vi "Get Oneof Fields.vi"(8 "error in (no error)":errorcluster, 11 "Message ref in":u64) -> (0 "error out":errorcluster, 2 "Field refs":u64[](array[numeric]), 3 "Message ref out":u64)   [LabVIEW 2019, in "gRPC Template Creation Utility.lvlib"]
uses:
  gRPC Template Creation Utility.lvlib
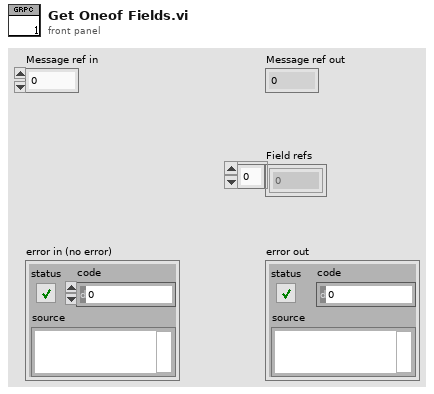
[diagram p1: front panel]
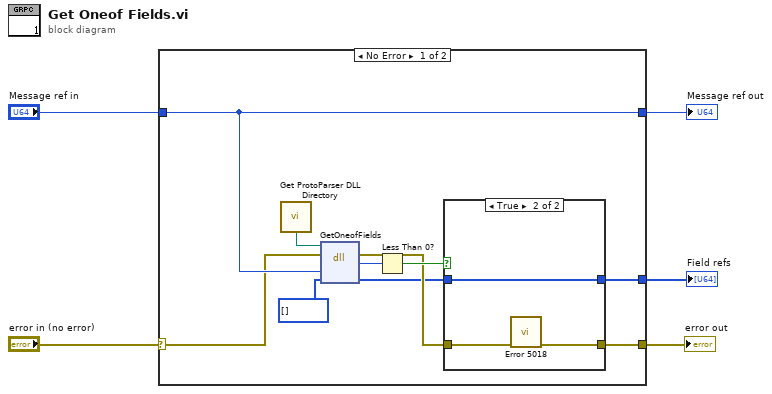
[diagram p0: block diagram]
diagram:
  n1 = case shown="No Error" "error in (no error)" {
    selector: "error in (no error)" -> [w12 w21]
    tunnel: "Message ref in" -> [w13 w22]
    tunnel: [w7 _] -> w4
    tunnel: [w13 w22] -> w3
    tunnel: [w6 w21] -> w1
    frame No Error {
      n2 = call "Get ProtoParser DLL Directory.vi"() -> ("Proto Parser Directory"=w14:path)
      n3 = dll-call lib="C:/Source/grpc-labview/build/Debug/labview_grpc_generator.dll" fn="GetOneofFields"(path in=w14, error in=w12, "message"=w13, "fieldInfo"=u64[] []) -> (error out=w9:errorcluster, "return type"=w11:i32, "fieldInfo"=w8:u64[])  [unwired: 2 in, 1 out]
      n4 = Less Than 0?(x=w11) -> (x < 0?=w10:bool)
      n5 = case shown="True" w10 {
        tunnel: w9 -> [w16 w20]
        tunnel: w8 -> [w17 w19]
        tunnel: [w17 w19] -> w7
        tunnel: [w16 w18] -> w6
        frame False {
        }
        frame True {
          n6 = call "Error 5018.vi"("error in (no error)"=w20) -> ("error out"=w18:errorcluster)  [unwired: 10 in]
        }
      }
    }
    frame Error {
    }
  }
  "Field refs" <- w4
  "Message ref out" <- w3
  "error out" <- w1
